vi "VCS Extract Channel Data Vector.vi"(0 "axis in":cluster{"keyHandle":u32, "nodeId":u16}={"keyHandle"=0, "nodeId"=1}, 5 "data buffer":T1, 7 "channelNumber":u8, 9 "vectorSize":u32, 11 "error in (no error)":errorcluster, 12 "objectSize":u8) -> (4 "axis out":cluster{"keyHandle":u32, "nodeId":u16}={"keyHandle"=0, "nodeId"=1}, 8 "data vector":u8[](array[numeric]), 15 "error out":errorcluster)   [LabVIEW 2019, in "maxonEPOS.lvlib"]
doc: "<B>VCS_ExtractChannelDataVector</B> returns the vector of one data channel."
uses:
  Examples/maxonEPOS.lvlib
  Resources/EposCmd.dll
  Resources/EposCmd64.dll
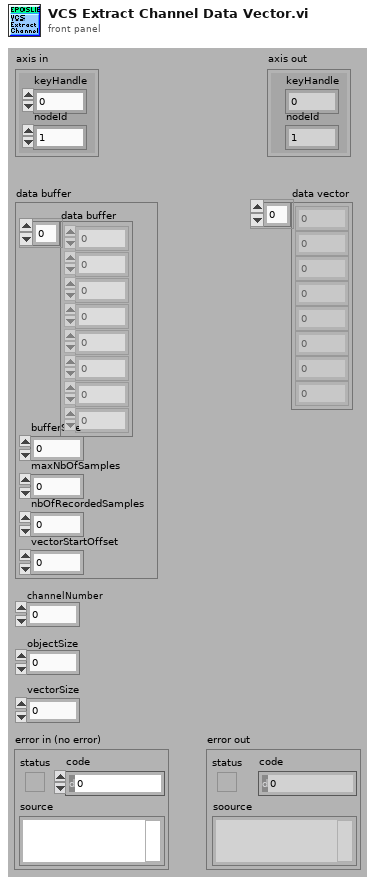
[diagram p1: front panel]
types:
  T1 = cluster{"bufferSize":u32, "vectorStartOffset":u16, "maxNbOfSamples":u16, "nbOfRecordedSamples":u16, "data buffer":u8[]}
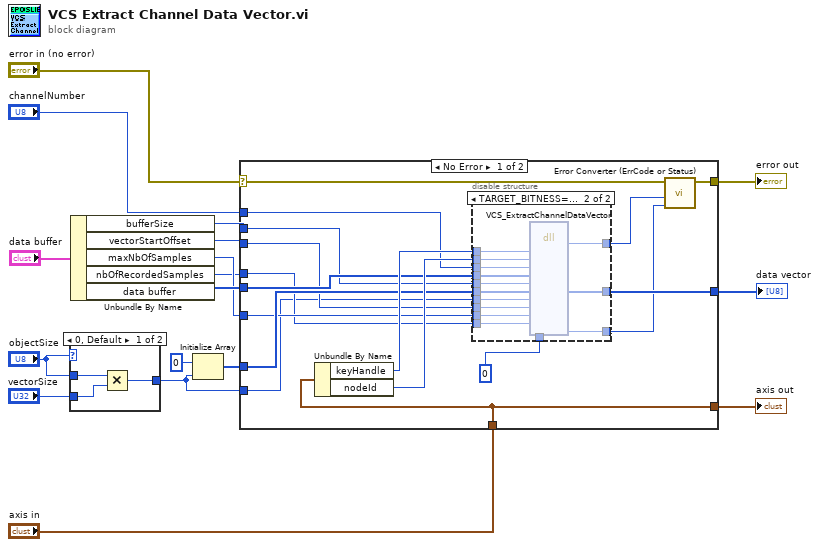
[diagram p0: block diagram]
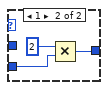
[diagram p2: hidden frame]
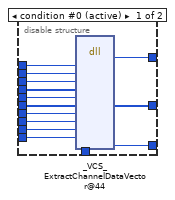
[diagram p3: hidden frame]
diagram:
  n1 = case shown="0, Default" "objectSize" {
    tunnel: [w20 w22] -> w3
    tunnel: "vectorSize" -> [w19 w21]
    tunnel: "objectSize" -> [w18 _]
    frame 0, Default {
      n2 = Multiply(x=w18, y=w19) -> (x*y=w20:u32)
    }
    frame 1 {
      n3 = Multiply(x=u32 2, y=w21) -> (x*y=w22:u32)
    }
  }
  n4 = Unbundle By Name("data buffer") -> ("bufferSize"=w7:u32, "vectorStartOffset"=w6:u16, "maxNbOfSamples"=w5:u16, "nbOfRecordedSamples"=w4:u16, "data buffer"=w8:u8[])
  n5 = Initialize Array(u8 0, w3) -> (w10:u8[])
  n6 = case shown="No Error" "error in (no error)" {
    selector: "error in (no error)" -> [w38 w70]
    tunnel: "axis in" -> [w40 w71]
    tunnel: [w40 w71] -> w16
    tunnel: [w39 w70] -> w15
    tunnel: [w37 w69] -> w11
    tunnel: "channelNumber" -> [w31 _]
    tunnel: w10 -> [w30 w69]
    tunnel: w8 -> [w29 _]
    tunnel: w7 -> [w28 _]
    tunnel: w6 -> [w27 _]
    tunnel: w5 -> [w26 _]
    tunnel: w4 -> [w25 _]
    tunnel: w3 -> [w24 _]
    frame No Error {
      n7 = Unbundle By Name(w40) -> ("keyHandle"=w35:u32, "nodeId"=w34:u16)
      n8 = disable-structure shown="TARGET_BITNESS==64" {
        disable-tunnel: [w54 w68] -> w37
        disable-tunnel: u32 0 ("pErrorCode") -> [w53 w67]
        disable-tunnel: w35 -> [w52 w66]
        disable-tunnel: w34 -> [w51 w65]
        disable-tunnel: [w50 w64] -> w33
        disable-tunnel: [w49 w63] -> w32
        disable-tunnel: w31 -> [w48 w62]
        disable-tunnel: w30 -> [w47 w61]
        disable-tunnel: w29 -> [w46 w60]
        disable-tunnel: w28 -> [w45 w59]
        disable-tunnel: w27 -> [w44 w58]
        disable-tunnel: w26 -> [w43 w57]
        disable-tunnel: w25 -> [w42 w56]
        disable-tunnel: w24 -> [w41 w55]
        frame condition #0 (active) {
          n9 = dll-call lib="C:/workspace/project/scancon/sw/SSI_Tool/InstrumentsInterfaces/Motordriver/maxon EPOS/Resources/EposCmd.*" fn="_VCS_ExtractChannelDataVector@44" ("VCS_ExtractChannelDataVector")("KeyHandle"=w52, "NodeId"=w51, "ChannelNumber"=w48, "pDataBuffer"=w46, "BufferSize"=w45, "pDataVector"=w47, "VectorSize"=w41, "VectorStartOffset"=w44, "MaxNbOfSamples"=w43, "NbOfRecordedSamples"=w42, "pErrorCode"=w53) -> ("Rückgabetyp"=w50:i32, "pDataVector"=w54:u8[], "pErrorCode"=w49:u32)  [unwired: 12 in, 2 out]
        }
        frame condition #1 {
          n10 = dll-call lib="C:/setup/Resources/EposCmd64.*" fn="VCS_ExtractChannelDataVector"("KeyHandle"=w66, "NodeId"=w65, "ChannelNumber"=w62, "pDataBuffer"=w60, "BufferSize"=w59, "pDataVector"=w61, "VectorSize"=w55, "VectorStartOffset"=w58, "MaxNbOfSamples"=w57, "NbOfRecordedSamples"=w56, "pErrorCode"=w67) -> ("Rückgabetyp"=w64:i32, "pDataVector"=w68:u8[], "pErrorCode"=w63:u32)  [unwired: 12 in, 2 out]
        }
      }
      n11 = call "Error Converter (ErrCode or Status).vi"("error code"=w32, "return type"=w33, "error in (no error)"=w38) -> ("error out"=w39:errorcluster)  [unwired: 7 in]
    }
    frame Error {
    }
  }
  "error out" <- w15
  "axis out" <- w16
  "data vector" <- w11
